vi "John simple relay switch.vi"() -> ()   [LabVIEW 2009]
uses:
  <vilib>/DAQmx/create/channels.llb/DAQmx Create Channel (DO-Digital Output).vi
  <vilib>/Platform/TimedLoop/XDataNode/XDataNode.xnode
  <vilib>/Platform/TimedLoop/XDataNode/loadlvalarms.vi
  <vilib>/Platform/TimedLoop/XDataNode/timing_clust.ctl
  <vilib>/Platform/TimedLoop/XDataNode/nitl_modes.ctl
  <vilib>/Platform/TimedLoop/XDataNode/wakeup.ctl
  <vilib>/Platform/TimedLoop/XDataNode/XDNodeRunTimeDep.lvlib
panel:
  in  "Wait for":dbl[unit]
  in  "stop":bool
  in  "Period":i64=1000
  out "counter":i8
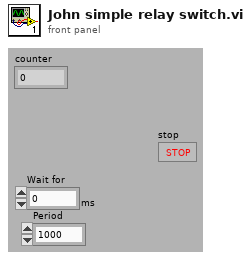
[diagram p1: front panel]
types:
  T1 = typedef "XDNodeRunTimeDep.lvlib/timing_clust.ctl" = cluster{"Expected End [f-1]":u64, "Actual End [f-1]":u64, "Finished Late? [f-1]":bool, "Expected End [i-1]":u64, "Actual End [i-1]":u64, "Finished Late? [i-1]":bool, "Expected Start [i]":u64, "Actual Start [i]":u64, "Expected Start [f]":u64, "Actual Start [f]":u64, "Source Name":string, "Structure Name":string, "Period":i64, "Deadline":i64, "Offset":i64, "Start":i64, "Priority":i32, "Timeout":i32, "Mode":T2, "Wakeup Reason":T3, "Error":errorcluster, "Source Type":string, "Secondary Source Type":string, "Global End Time":u64, "Global Start Time":u64, "Frame Duration":u64, "Iteration Duration":u64, "Assigned CPU":i32, "I/O Scan Engine Mode":u32}
  T2 = typedef "XDNodeRunTimeDep.lvlib/nitl_modes.ctl" = enum32{"No Change", "Process missed periods, maintain original phase", "Discard missed periods, maintain original phase", "Process missed periods, ignore original phase", "Discard missed periods, ignore original phase"}
  T3 = typedef "XDNodeRunTimeDep.lvlib/wakeup.ctl" = enum32{"Normal", "Aborted", "Asynchronous wakeup", "Timing source error", "Timed loop error", "Timeout"}
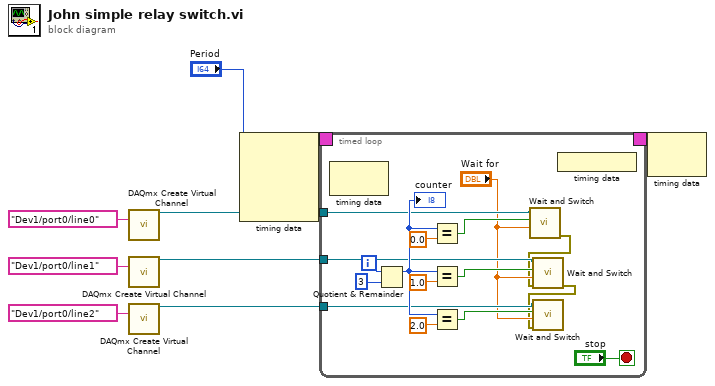
[diagram p0: block diagram]
diagram:
  n1 = call-poly <vilib>:"DAQmx Create Virtual Channel.vi"("lines"=tag "Dev1/port0/line0") -> ("task out"=w6:refnum<k21>)  [unwired: 5 in, 9 out]
  n2 = call-poly <vilib>:"DAQmx Create Virtual Channel.vi"("lines"=tag "Dev1/port0/line1") -> ("task out"=w5:refnum<k21>)  [unwired: 5 in, 9 out]
  n3 = call-poly <vilib>:"DAQmx Create Virtual Channel.vi"("lines"=tag "Dev1/port0/line2") -> ("task out"=w4:refnum<k21>)  [unwired: 5 in, 9 out]
  n4 = node-c288("Period") -> (w3:T1)  [unwired: 3 out]
  n5 = timed-loop {
    timing: w3 -> [_]
    timing-out: [_] -> w2
    tunnel: w4 -> [w13]
    tunnel: w5 -> [w18]
    tunnel: w6 -> [w17]
    i -> [w21]
    stop <- "stop" stop-if-true
    n6 = node-c288() -> ()  [unwired: 2 out]
    n7 = Quotient & Remainder(x=w21, y=3) -> (x-y*floor(x/y)=w20:i32)  [unwired: 1 out]
    "counter" <- w20
    n8 = Equal?(x=w20, y=0.0) -> (x = y?=w16:bool)
    n9 = Equal?(x=w20, y=1.0) -> (x = y?=w15:bool)
    n10 = Equal?(x=w20, y=2.0) -> (x = y?=w14:bool)
    n11 = call "Wait and Switch.vi"("Wait for"="Wait for", "Switch to"=w16, "task in"=w17) -> ("error out"=w11:errorcluster)  [unwired: 1 in, 7 out]
    n12 = call "Wait and Switch.vi"("error in"=w11, "Wait for"="Wait for", "Switch to"=w15, "task in"=w18) -> ("error out"=w10:errorcluster)  [unwired: 7 out]
    n13 = call "Wait and Switch.vi"("error in"=w10, "Wait for"="Wait for", "Switch to"=w14, "task in"=w13) -> ()  [unwired: 8 out]
    n14 = node-c288() -> ()  [unwired: 1 out]
  }
  n15 = node-c288(w2) -> ()  [unwired: 1 out]
